vi "GetProviderName.vi"(0 "ClassWriterNative in":refnum<class "ClassWriterNative.lvclass">, 5 "error in (no error)":errorcluster) -> (14 "ClassWriterNative out":refnum<class "ClassWriterNative.lvclass">, 15 "ProviderName":string, 17 "TranslatedProviderName":string, 18 "ShortName(Could be used in for INI Sections)":string, 19 "error out":errorcluster)   [LabVIEW 2020, in "ClassWriterNative.lvclass"]
uses:
  <resource>/Framework/Providers/Open_GDS/ClassProviders/Provider_LvNativeClass/ClassWriterNative_class/ClassWriterNative.lvclass
  <resource>/Framework/Providers/Open_GDS/ClassProviders/Provider_LvNativeClass/LvNativeProviderName.ctl
  <resource>/Framework/Providers/Open_GDS/ClassProviders/Provider_LvNativeClass/ClassWriterNative_class/ClassWriterNative.lvclass/ClassWriterNative.ctl
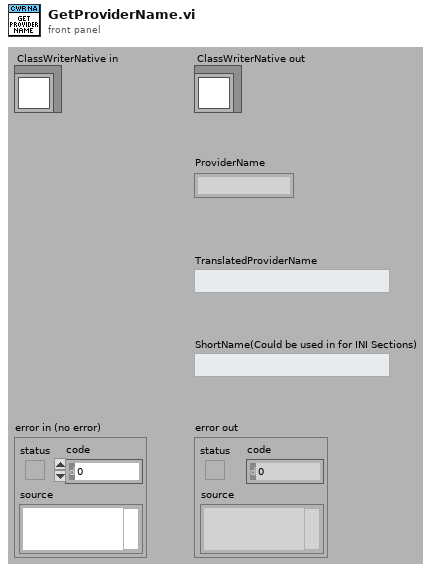
[diagram p1: front panel]
types:
  T1 = typedef "LvNativeProviderName.ctl" = enum16{"Endevo LabVIEW Native"}
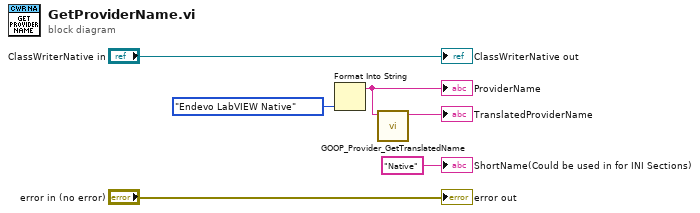
[diagram p0: block diagram]
diagram:
  n1 = Format Into String(LvNativeProviderName."Endevo LabVIEW Native" ("ProviderName")) -> (resulting string=w2:string)  [unwired: 3 in, 1 out]
  "ProviderName" <- w2
  n2 = call <resource>:"GOOP_Provider_GetTranslatedName.vi"("ProviderName"=w2) -> ("TranslatedName"=→"TranslatedProviderName":string)  [unwired: 10 in]
  "ClassWriterNative out" <- "ClassWriterNative in"
  "error out" <- "error in (no error)"
  "ShortName(Could be used in for INI Sections)" <- "Native" ("ClassType")
